vi "queue dequeue.vi"() -> ()   [LabVIEW 2012]
panel:
  in  "stop 2":bool
  in  "stop":bool
  out "Dequed data 2":dbl
  out "Dequed data":dbl
  in  "Master 3":bool
  in  "Queued 2":dbl
  in  "Master 4":bool
  in  "Queued 1":dbl
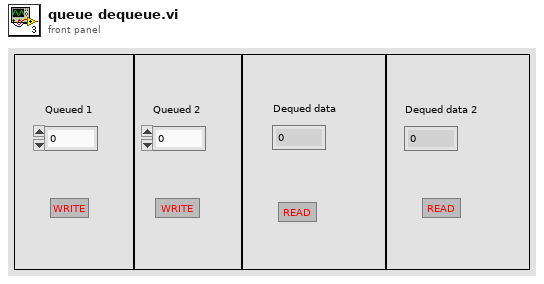
[diagram p1: front panel]
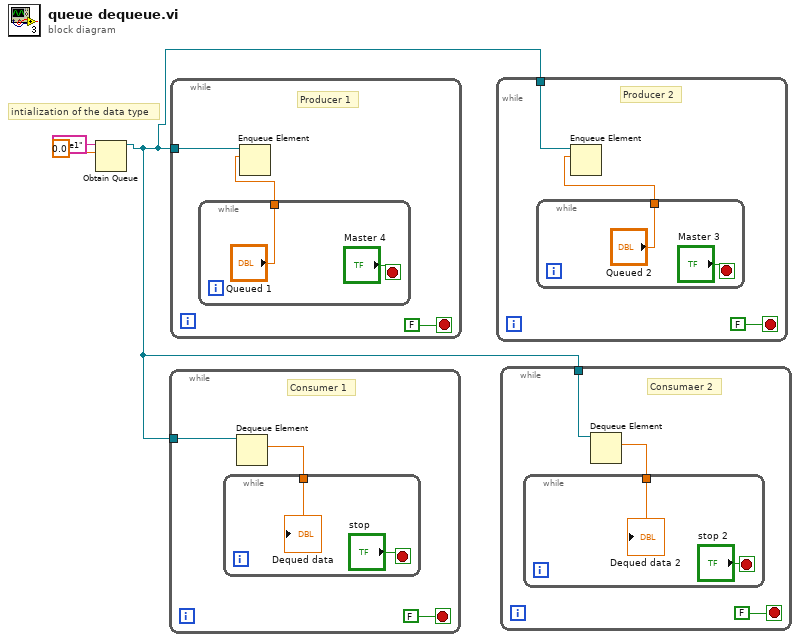
[diagram p0: block diagram]
diagram:
  # "intialization of the data type"
  n1 = Obtain Queue(name (unnamed)="que1", element data type=0.0 ("Numeric 2")) -> (queue out=w2:refnum<queue>)  [unwired: 3 in, 2 out]
  n2 = while {
    tunnel: w2 -> [w5]
    stop <- FALSE stop-if-true
    # "Consumer 1"
    n3 = Dequeue Element(queue=w5) -> (element=w4:dbl)  [unwired: 2 in, 3 out]
    n4 = while {
      tunnel: w4 -> [w8]
      stop <- "stop" stop-if-true
      "Dequed data" <- w8
    }
  }
  n5 = while {
    tunnel: w2 -> [w10]
    stop <- FALSE stop-if-true
    # "Producer 1"
    n6 = while {
      tunnel: ["Queued 1"] -> w9
      stop <- "Master 4" stop-if-true
    }
    n7 = Enqueue Element(queue=w10, element=w9) -> ()  [unwired: 2 in, 3 out]
  }
  n8 = while {
    tunnel: w2 -> [w15]
    stop <- FALSE stop-if-true
    # "Producer 2"
    n9 = while {
      tunnel: ["Queued 2"] -> w14
      stop <- "Master 3" stop-if-true
    }
    n10 = Enqueue Element(queue=w15, element=w14) -> ()  [unwired: 2 in, 3 out]
  }
  n11 = while {
    tunnel: w2 -> [w20]
    stop <- FALSE stop-if-true
    # "Consumaer 2"
    n12 = Dequeue Element(queue=w20) -> (element=w19:dbl)  [unwired: 2 in, 3 out]
    n13 = while {
      tunnel: w19 -> [w23]
      stop <- "stop 2" stop-if-true
      "Dequed data 2" <- w23
    }
  }
